vi "Make VI Param(Profile Info).vi"(1 "pProfileInfo":T1) -> (0 "Profile Info":T2)   [LabVIEW 2015, in "KEYENCE LJ-X8000A.lvlib"]
uses:
  KEYENCE LJ-X8000A.lvlib
  Public/Clusters/Profile Info.ctl
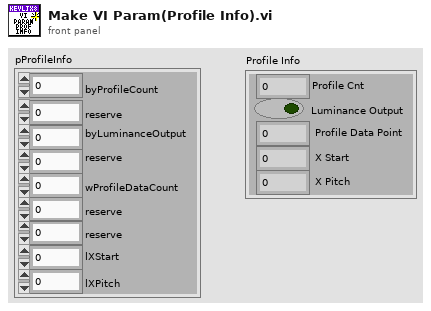
[diagram p1: front panel]
types:
  T1 = cluster{"byProfileCount":u8, "reserve":u8, "byLuminanceOutput":u8, "reserve":u8, "wProfileDataCount":u16, "reserve":u8, "reserve":u8, "lXStart":i32, "lXPitch":i32}
  T2 = typedef "KEYENCE LJ-X8000A.lvlib/Profile Info.ctl" = cluster{"Profile Cnt":u8, "Luminance Output":bool, " Profile Data Point":u16, " X Start":i32, " X Pitch":i32}
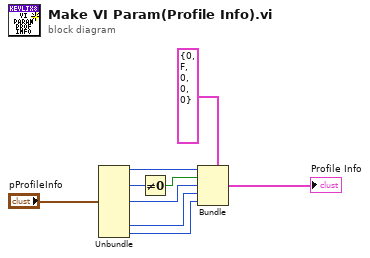
[diagram p0: block diagram]
diagram:
  n1 = Unbundle("pProfileInfo") -> ("byProfileCount"=w5:u8, "byLuminanceOutput"=w1:u8, "wProfileDataCount"=w7:u16, "lXStart"=w8:i32, "lXPitch"=w9:i32)  [unwired: 4 out]
  n2 = Not Equal To 0?(x=w1) -> (x != 0?=w6:bool)
  n3 = Bundle(cluster=T2 {"Profile Cnt"=0, "Luminance Output"=FALSE, " Profile Data Point"=0, " X Start"=0, " X Pitch"=0} ("Profile Info"), "Profile Cnt"=w5, "Luminance Output"=w6, "Profile Data Point"=w7, "X Start"=w8, "X Pitch"=w9) -> (→"Profile Info":T2)
